vi "Treshhol 2D Array.vi"(9 "Invert low X":bool=TRUE, 10 "X row":i32, 11 "Array":dbl[][](array[numeric])) -> (2 "Output high array":dbl[][](array[numeric]), 3 "Output low array":dbl[][](array[numeric]))   [LabVIEW 2025]
panel:
  out "Split and binned +B and -B":cluster{dbl[], dbl[]}[](graph) caption="XY Graph"
  in  "threshold":dbl
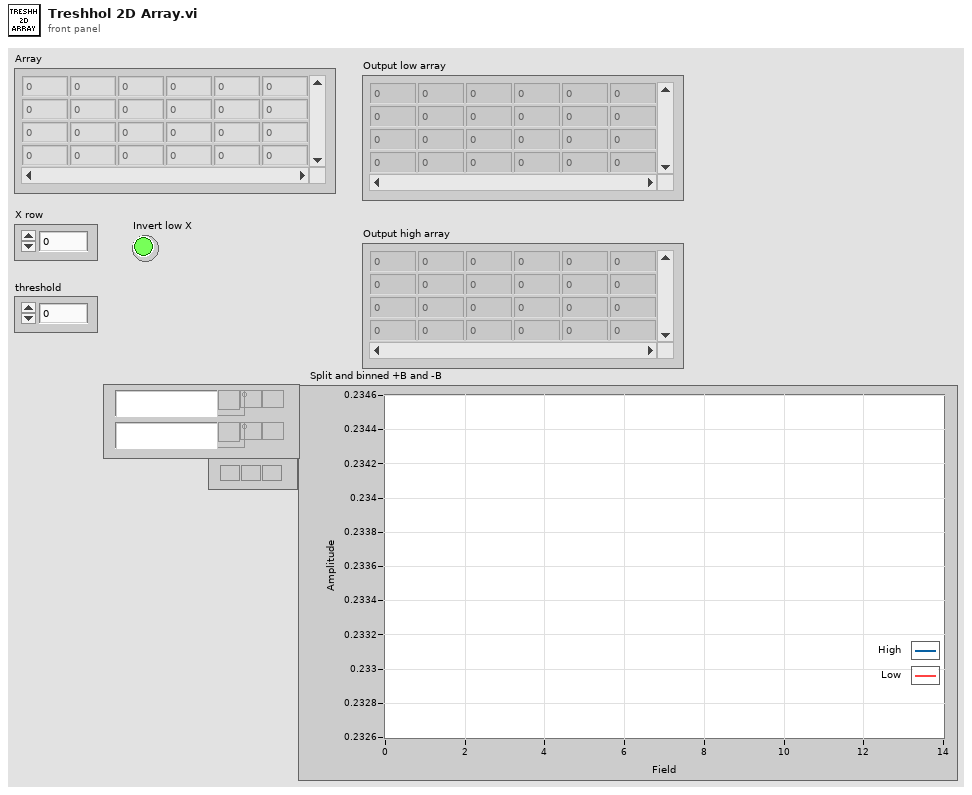
[diagram p1: front panel]
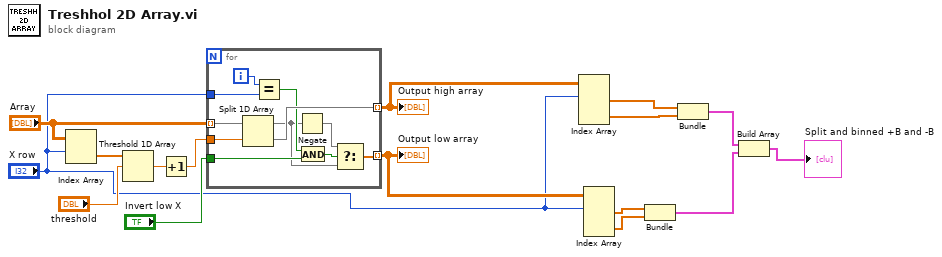
[diagram p0: block diagram]
diagram:
  n1 = Index Array(array="Array", index (row)="X row") -> (element=w15:dbl[])  [unwired: 1 in]
  n2 = Threshold 1D Array(2:"threshold", 3:w15) -> (0:w13:dbl)  [unwired: 1 in]
  n3 = Increment(x=w13) -> (x+1=w12:dbl)
  n4 = for {
    tunnel: "Array" -> [w27] mode=indexing
    tunnel: [w19] -> w9 mode=indexing
    tunnel: [w26] -> w10 mode=indexing
    tunnel: w12 -> [w25]
    tunnel: "X row" -> [w18]
    tunnel: "Invert low X" -> [w23]
    i -> [w17]
    n5 = Split 1D Array(array=w27, index=w25) -> (first subarray=w20:dbl[], second subarray=w26:dbl[])
    n6 = Equal?(x=w17, y=w18) -> (x = y?=w24:bool)
    n7 = Negate(x=w20) -> (-x=w22:dbl[])
    n8 = And(x=w24, y=w23) -> (x .and. y?=w21:bool)
    n9 = Select(t=w22, s=w21, f=w20) -> (s? t:f=w19:dbl[])
  }
  "Output low array" <- w9
  "Output high array" <- w10
  n10 = Index Array(array=w10, index (row) #1="X row") -> (element #1=w7:dbl[], element #2=w6:dbl[])  [unwired: 3 in]
  n11 = Index Array(array=w9, index (row) #1="X row") -> (element #1=w4:dbl[], element #2=w5:dbl[])  [unwired: 3 in]
  n12 = Bundle(w4, w5) -> (w2:cluster{dbl[], dbl[]})  [unwired: 1 in]
  n13 = Bundle(w7, w6) -> (w3:cluster{dbl[], dbl[]})  [unwired: 1 in]
  n14 = Build Array(w3, w2) -> (→"Split and binned +B and -B":cluster{dbl[], dbl[]}[])
